vi "offsets.vi"() -> ()   [LabVIEW 2015, in "LVJSON.lvlib" / "Set Object Parameters.xnode"]
uses:
  Set Object Parameters.xnode
panel:
  in  "Tab Control":enum32{"offsets"}(tab)
  in  "row width":i16=150
  in  "row height":i16=18
  in  "header size":i16=32
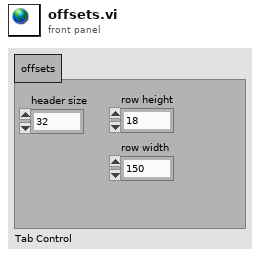
[diagram p1: front panel]
diagram:
